vi "Begin.vi"(11 "Image Size":T1=enum."160x120") -> (0 "error out":errorcluster)   [LabVIEW 2011]
doc: "Called before other user functions, this VI is expected to open initial I/O refnums, load in file data, and do all program initialization. Notice that the <B>error out</B> terminal is simply used for data flow. Wiring it to other structures or subVIs ensures that this VI runs first."
uses:
  <vilib>/Rock Robotics/WPI/Camera/WPI_CameraImageSize.ctl
  <vilib>/Rock Robotics/WPI/Camera/WPI_CameraWhite Balance Values.ctl
  <vilib>/Rock Robotics/WPI/Camera/WPI_CameraExposure Values.ctl
  <vilib>/Rock Robotics/WPI/Camera/WPI_CameraFrameRate.ctl
  <vilib>/Rock Robotics/SystemInterfaces/DIO/FPGA_DIOPWMChannel.ctl
  <vilib>/Rock Robotics/SystemInterfaces/Typedef/FPGA_TypedefDigitalModule.ctl
  <vilib>/Rock Robotics/SystemInterfaces/DIO/FPGA_DIOChannel.ctl
  <vilib>/Rock Robotics/WPI/Encoder/WPI_EncoderType.ctl
  <vilib>/Rock Robotics/SystemInterfaces/Typedef/FPGA_TypedefAnalogModule.ctl
  <vilib>/Rock Robotics/SystemInterfaces/AI/FPGA_AIChannel.ctl
  <vilib>/Rock Robotics/SystemInterfaces/DIO/FPGA_DIORelayChannel.ctl
  <vilib>/Rock Robotics/WPI/Joystick/WPI_JoystickDeviceEnum.ctl
  <vilib>/Rock Robotics/WPI/RobotDrive/WPI_RobotDriveOpen4MotorWithVictor.vi
  <vilib>/Rock Robotics/WPI/MotorControl/WPI_MotorControlOpen Victor.vi
  <vilib>/Rock Robotics/WPI/Counter/WPI_CounterDigitalInputToDigitalSource.vi
panel:
  in  "Image Size 2":T1=enum."160x120"
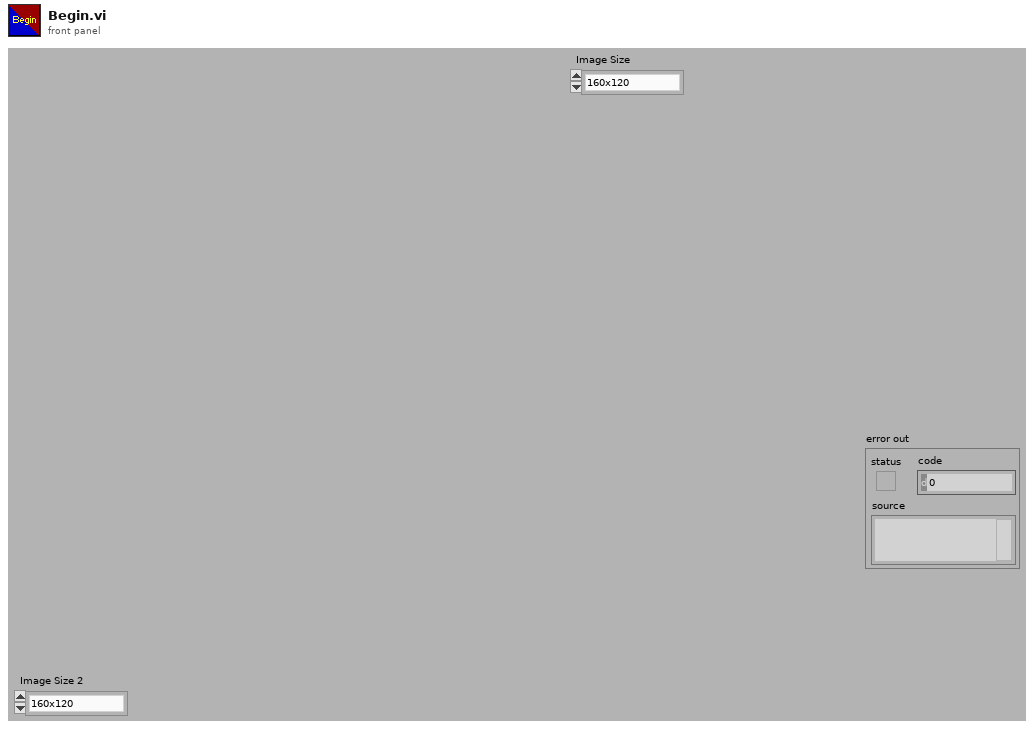
[diagram p1: front panel]
types:
  T1 = typedef "WPI_CameraImageSize.ctl" = enum16{"640x480", "320x240", "160x120"}
  T2 = typedef "FPGA_DIOChannel.ctl" = enum8{"DIO 1", "DIO 2", "DIO 3", "DIO 4", "DIO 5", "DIO 6", "DIO 7", "DIO 8", "DIO 9", "DIO 10", "DIO 11", "DIO 12", "DIO 13", "DIO 14", "Invalid"}
  T3 = typedef "FPGA_TypedefDigitalModule.ctl" = enum16{"Digital Module 1", "Digital Module 2"}
  T4 = typedef "FPGA_DIORelayChannel.ctl" = enum8{"Relay 1", "Relay 2", "Relay 3", "Relay 4", "Relay 5", "Relay 6", "Relay 7", "Relay 8", "Invalid"}
  T5 = typedef "WPI_JoystickDeviceEnum.ctl" = enum16{"USB 1", "USB 2", "USB 3", "USB 4", "Kinect 1", "Kinect 2"}
  T6 = typedef "FPGA_DIOPWMChannel.ctl" = enum8{"PWM 1", "PWM 2", "PWM 3", "PWM 4", "PWM 5", "PWM 6", "PWM 7", "PWM 8", "PWM 9", "PWM 10", "Invalid"}
  T7 = typedef "FPGA_AIChannel.ctl" = enum8{"AI 1", "AI 2", "AI 3", "AI 4", "AI 5", "AI 6", "AI 7", "AI 8", "Invalid"}
  T8 = typedef "FPGA_TypedefAnalogModule.ctl" = enum16{"Analog Module 1", "Analog Module 2"}
  T9 = typedef "WPI_EncoderType.ctl" = enum16{"1x", "2x", "4x"}
  T10 = typedef "WPI_CameraFrameRate.ctl" = u32
  T11 = typedef "WPI_CameraExposure Values.ctl" = enum16{"Auto", "Flicker-free 50 Hz", "Flicker-free 60 Hz", "Hold current"}
  T12 = typedef "WPI_CameraWhite Balance Values.ctl" = enum16{"Auto", "Fixed indoor", "Fixed outdoor 1", "Fixed outdoor 2", "Fixed fluorescent 1", "Fixed fluorescent 2", "Hold current"}
  T13 = typedef "WPI_MotorControlDeviceRef.ctl" = cluster{"DeviceStatus":errorcluster, "Type":enum16{"PWM", "CAN"}, "PWM":cluster{"Digital Module":T3, "PWM Channel":T6, "DeadBand":T14}, "CAN":cluster{"Device Number":u8, "Control Mode":T15, "Semaphore":T16, "Max Vout":dbl}, "Invert":bool, "TransformRef":T17, "InvTransformRef":T17}
  T14 = typedef "WPI_PWMDeadband.ctl" = cluster{"Name":string, "maxPositivePwm":i32, "minPositivePwm":i32, "centerPwm":i32, "maxNegativePwm":i32, "minNegativePwm":i32, "angularRange":u16}
  T15 = typedef "WPI_CANJaguar_ControlMode.ctl" = enum8{"Percent VBus", "Current", "Speed", "Position", "Voltage"}
  T16 = typedef "Semaphore RefNum" = refnum<k1>
  T17 = typedef "WPI_PWMTransform_ConPane.ctl" = refnum<vi>
  T18 = typedef "WPI_RobotDriveDevRef.ctl" = cluster{"DevStatus":errorcluster, "Motors[]":T13[], "Square Inputs":bool, "Max Output":dbl, "Isochronous":bool}
  T19 = typedef "WPI_CameraDevRef.ctl" = cluster{"Camera Address":string, "CameraStatus":errorcluster, "Acquire Image Notifier":refnum<notifier>}
  T20 = typedef "WPI_DigitalInputDevRef.ctl" = cluster{"DevStatus":errorcluster, "DIO Channel":T2, "Digital Module":T3}
  T21 = typedef "FPGA_CounterEncoderSourceConvertionLVSourceType.ctl" = cluster{"DevStatus":errorcluster, "AnalogTriggerMode?":bool, "DigitalMode":cluster{"Digital Module":T3, "DIO Channel":T22}, "AnalogTriggerMode":cluster{"AnalogTriggerIndex":T23, "OutputType":T24}}
  T22 = typedef "FPGA_DIODigitalSourceChannel.ctl" = enum8{"DIO 1", "DIO 2", "DIO 3", "DIO 4", "DIO 5", "DIO 6", "DIO 7", "DIO 8", "DIO 9", "DIO 10", "DIO 11", "DIO 12", "DIO 13", "DIO 14", "Disabled"}
  T23 = typedef "FPGA_AnalogTriggerIndex.ctl" = enum8{"Trig 0", "Trig 1", "Trig 2", "Trig 3", "Trig 4", "Trig 5", "Trig 6", "Trig 7", "Invalid"}
  T24 = typedef "FPGA_AnalogTriggerOutType.ctl" = enum16{"InWindow", "TriggerState", "Rising", "Falling"}
  T25 = typedef "WPI_AnalogChannelDevRef.ctl" = cluster{"DevStatus":errorcluster, "Analog Module":T8, "Analog Channel":T7}
  T26 = typedef "WPI_JoystickDevRef.ctl" = cluster{"Device":T5}
  T27 = typedef "WPI_RelayDevRef.ctl" = cluster{"DevStatus":errorcluster, "Relay Channel":T4, "Digital Module":T3, "Relay Direction":T28}
  T28 = typedef "WPI_RelayDirection.ctl" = enum16{"Both directions", "Forward only", "Reverse only"}
  T29 = typedef "WPI_EncoderDevRef.ctl" = cluster{"DevStatus":errorcluster, "EncoderIndex":T30, "CounterIndex":T31, "DistancePerCount":dbl, "Decoding Type":T9}
  T30 = typedef "FPGA_EncoderIdx.ctl" = enum8{"Enc 0", "Enc 1", "Enc 2", "Enc 3", "Invalid"}
  T31 = typedef "FPGA_CounterCtrSystemIndex.ctl" = enum8{"Ctr 0", "Ctr 1", "Ctr 2", "Ctr 3", "Ctr 4", "Ctr 5", "Ctr 6", "Ctr 7", "Invalid"}
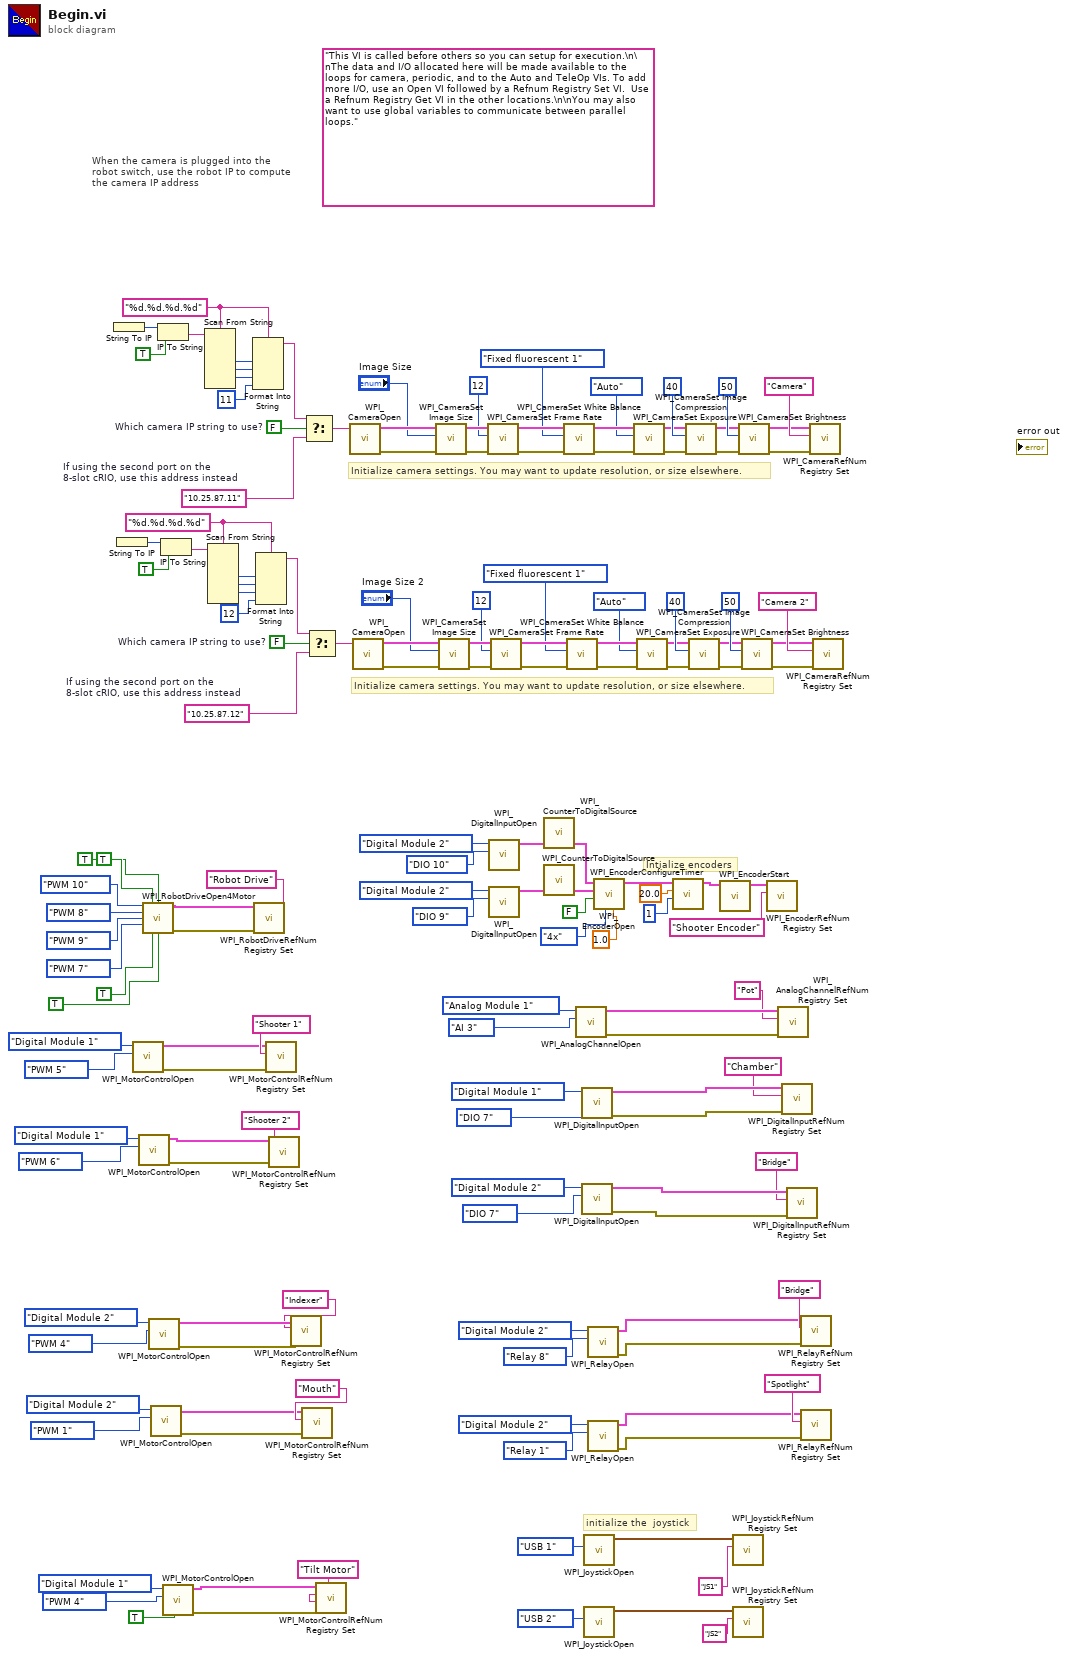
[diagram p0: block diagram]
diagram:
  w86 = FALSE  # Which camera IP string to use?
  w90 = "%d.%d.%d.%d" ("format string")
  w87 = "10.25.87.12"  # If using the second port on the 8-slot cRIO, use this address instead
  w119 = FALSE  # Which camera IP string to use?
  w123 = "%d.%d.%d.%d" ("format string")
  (unwired) "This VI is called before others so you can setup for execution.\n\nThe data and I/O allocated here will be made available to the loops for camera, periodic, and to the Auto and TeleOp VIs. To add more I/O, use an Open VI followed by a Refnum Registry Set VI.  Use a Refnum Registry Get VI in the other locations.\n\nYou may also want to use global variables to communicate between parallel loops."
  w120 = "10.25.87.11"  # If using the second port on the 8-slot cRIO, use this address instead
  # "initialize the  joystick"
  # "Intialize encoders"
  # "Initialize camera settings. You may want to update resolution, or size elsewhere."
  # "When the camera is plugged into the\nrobot switch, use the robot IP to compute\nthe camera IP address"
  # "Initialize camera settings. You may want to update resolution, or size elsewhere."
  n1 = String To IP() -> (0:w130:u32)  [unwired: 1 in]
  n2 = String To IP() -> (0:w97:u32)  [unwired: 1 in]
  n3 = call-poly <vilib>:"WPI_MotorControlOpen.vi"("PWM Channel"=FPGA_DIOPWMChannel."PWM 5", "Digital Module (Module 1)"=FPGA_TypedefDigitalModule."Digital Module 1") -> ("error out"=w69:errorcluster, "MotorControlDeviceRef"=w70:T13)  [unwired: 8 in]
  n4 = call-poly <vilib>:"WPI_MotorControlOpen.vi"("PWM Channel"=FPGA_DIOPWMChannel."PWM 6", "Digital Module (Module 1)"=FPGA_TypedefDigitalModule."Digital Module 1") -> ("error out"=w67:errorcluster, "MotorControlDeviceRef"=w68:T13)  [unwired: 8 in]
  n5 = call-poly <vilib>:"WPI_RobotDriveOpen4Motor.vi"("Rear Left Motor"=FPGA_DIOPWMChannel."PWM 10", "Rear Left Motor Inverted"=TRUE, "Rear Right Motor Inverted"=TRUE, "Rear Right Motor"=FPGA_DIOPWMChannel."PWM 8", "Front Left Motor"=FPGA_DIOPWMChannel."PWM 9", "Front Right Motor"=FPGA_DIOPWMChannel."PWM 7", "Front Left Motor Inverted"=TRUE, "Front Right Motor Inverted"=TRUE) -> ("RobotDriveDevRef"=w12:T18, "error out"=w11:errorcluster)  [unwired: 6 in]
  n6 = call-poly <vilib>:"WPI_MotorControlOpen.vi"("PWM Channel"=FPGA_DIOPWMChannel."PWM 4", "Digital Module (Module 1)"=FPGA_TypedefDigitalModule."Digital Module 2") -> ("error out"=w20:errorcluster, "MotorControlDeviceRef"=w21:T13)  [unwired: 8 in]
  n7 = call-poly <vilib>:"WPI_MotorControlOpen.vi"("PWM Channel"=FPGA_DIOPWMChannel."PWM 1", "Digital Module (Module 1)"=FPGA_TypedefDigitalModule."Digital Module 2") -> ("error out"=w62:errorcluster, "MotorControlDeviceRef"=w63:T13)  [unwired: 8 in]
  n8 = IP To String(1:TRUE ("dot notation? (F)"), 2:w130) -> (0:w128:string)
  n9 = IP To String(1:TRUE ("dot notation? (F)"), 2:w97) -> (0:w95:string)
  n10 = call-poly <vilib>:"WPI_MotorControlOpen.vi"("Invert"=TRUE, "PWM Channel"=FPGA_DIOPWMChannel."PWM 4", "Digital Module (Module 1)"=FPGA_TypedefDigitalModule."Digital Module 1") -> ("error out"=w56:errorcluster, "MotorControlDeviceRef"=w57:T13)  [unwired: 7 in]
  n11 = Scan From String(format string=w123, input string=w128) -> (output 1=w127:i32, output 2=w126:i32, output 3=w125:i32)  [unwired: 7 in, 3 out]
  n12 = Scan From String(format string=w90, input string=w95) -> (output 1=w94:i32, output 2=w93:i32, output 3=w92:i32)  [unwired: 7 in, 3 out]
  n13 = Format Into String(format string=w123, w127, w126, w125, 11 ("Compression")) -> (resulting string=w121:string)  [unwired: 2 in, 1 out]
  n14 = call <vilib>:"WPI_RobotDriveRefNum Registry Set.vi"("error in (no error)"=w11, "refnum name"="Robot Drive", "RobotDriveDevRef"=w12) -> ()  [unwired: 7 in, 2 out]
  n15 = Format Into String(format string=w90, w94, w93, w92, 12 ("Compression")) -> (resulting string=w88:string)  [unwired: 2 in, 1 out]
  n16 = call <vilib>:"WPI_MotorControlRefNum Registry Set.vi"("error in (no error)"=w69, "refnum name"="Shooter 1", "MotorControlDevRef"=w70) -> ()  [unwired: 7 in, 2 out]
  n17 = call <vilib>:"WPI_MotorControlRefNum Registry Set.vi"("error in (no error)"=w67, "refnum name"="Shooter 2", "MotorControlDevRef"=w68) -> ()  [unwired: 7 in, 2 out]
  n18 = call <vilib>:"WPI_MotorControlRefNum Registry Set.vi"("error in (no error)"=w20, "refnum name"="Indexer", "MotorControlDevRef"=w21) -> ()  [unwired: 7 in, 2 out]
  n19 = call <vilib>:"WPI_MotorControlRefNum Registry Set.vi"("error in (no error)"=w62, "refnum name"="Mouth", "MotorControlDevRef"=w63) -> ()  [unwired: 7 in, 2 out]
  n20 = Select(t=w121, s=w119, f=w120) -> (s? t:f=w122:string)
  n21 = Select(t=w88, s=w86, f=w87) -> (s? t:f=w89:string)
  n22 = call <vilib>:"WPI_MotorControlRefNum Registry Set.vi"("error in (no error)"=w56, "refnum name"="Tilt Motor", "MotorControlDevRef"=w57) -> ()  [unwired: 7 in, 2 out]
  n23 = call <vilib>:"WPI_CameraOpen.vi"("Camera Address"=w122) -> ("error out"=w142:errorcluster, "CameraDevRef"=w143:T19)  [unwired: 1 in, 8 out]
  n24 = call <vilib>:"WPI_CameraOpen.vi"("Camera Address"=w89) -> ("error out"=w109:errorcluster, "CameraDevRef"=w110:T19)  [unwired: 1 in, 8 out]
  n25 = call <vilib>:"WPI_CameraSet Image Size.vi"("error in (no error)"=w142, "Image Size"="Image Size", "CameraDevRef"=w143) -> ("error out"=w141:errorcluster, "CameraDevRef Out"=w144:T19)  [unwired: 7 out]
  n26 = call <vilib>:"WPI_CameraSet Image Size.vi"("error in (no error)"=w109, "Image Size"="Image Size 2", "CameraDevRef"=w110) -> ("error out"=w108:errorcluster, "CameraDevRef Out"=w111:T19)  [unwired: 7 out]
  n27 = call <vilib>:"WPI_CameraSet Frame Rate.vi"("error in (no error)"=w141, "Frame Rate (fps)"=T10 12, "CameraDevRef"=w144) -> ("error out"=w140:errorcluster, "CameraDevRef Out"=w146:T19)  [unwired: 7 out]
  n28 = call <vilib>:"WPI_DigitalInputOpen.vi"("DIO Channel"=FPGA_DIOChannel."DIO 10", "Digital Module (Module 1)"=FPGA_TypedefDigitalModule."Digital Module 2") -> ("DigitalInputDevRef"=w53:T20)  [unwired: 8 in, 1 out]
  n29 = call <vilib>:"WPI_DigitalInputOpen.vi"("DIO Channel"=FPGA_DIOChannel."DIO 9", "Digital Module (Module 1)"=FPGA_TypedefDigitalModule."Digital Module 2") -> ("DigitalInputDevRef"=w49:T20)  [unwired: 8 in, 1 out]
  n30 = call <vilib>:"WPI_CameraSet Frame Rate.vi"("error in (no error)"=w108, "Frame Rate (fps)"=T10 12, "CameraDevRef"=w111) -> ("error out"=w107:errorcluster, "CameraDevRef Out"=w113:T19)  [unwired: 7 out]
  n31 = call-poly <vilib>:"WPI_CounterToDigitalSource.vi"("DigitalInputDevRef"=w53) -> ("Digital Source"=w52:T21)  [unwired: 6 in]
  n32 = call-poly <vilib>:"WPI_CounterToDigitalSource.vi"("DigitalInputDevRef"=w49) -> ("Digital Source"=w48:T21)  [unwired: 6 in]
  n33 = call <vilib>:"WPI_CameraSet White Balance.vi"("error in (no error)"=w140, "White Balance"=WPI_CameraWhite_Balance_Values."Fixed fluorescent 1", "CameraDevRef"=w146) -> ("error out"=w139:errorcluster, "CameraDevRef Out"=w145:T19)  [unwired: 7 out]
  n34 = call <vilib>:"WPI_CameraSet White Balance.vi"("error in (no error)"=w107, "White Balance"=WPI_CameraWhite_Balance_Values."Fixed fluorescent 1", "CameraDevRef"=w113) -> ("error out"=w106:errorcluster, "CameraDevRef Out"=w112:T19)  [unwired: 7 out]
  n35 = call <vilib>:"WPI_AnalogChannelOpen.vi"("Analog Channel"=FPGA_AIChannel."AI 3", "Analog Module (Module 1)"=FPGA_TypedefAnalogModule."Analog Module 1") -> ("error out"=w34:errorcluster, "AIDeviceRef"=w36:T25)  [unwired: 8 in]
  n36 = call <vilib>:"WPI_DigitalInputOpen.vi"("DIO Channel"=FPGA_DIOChannel."DIO 7", "Digital Module (Module 1)"=FPGA_TypedefDigitalModule."Digital Module 1") -> ("error out"=w29:errorcluster, "DigitalInputDevRef"=w31:T20)  [unwired: 8 in]
  n37 = call <vilib>:"WPI_DigitalInputOpen.vi"("DIO Channel"=FPGA_DIOChannel."DIO 7", "Digital Module (Module 1)"=FPGA_TypedefDigitalModule."Digital Module 2") -> ("error out"=w1:errorcluster, "DigitalInputDevRef"=w3:T20)  [unwired: 8 in]
  n38 = call <vilib>:"WPI_JoystickOpen.vi"("JoystickDevice"=WPI_JoystickDeviceEnum."USB 1") -> ("JoystickDevRef"=w16:T26)  [unwired: 10 out]
  n39 = call <vilib>:"WPI_JoystickOpen.vi"("JoystickDevice"=WPI_JoystickDeviceEnum."USB 2") -> ("JoystickDevRef"=w15:T26)  [unwired: 10 out]
  n40 = call <vilib>:"WPI_RelayOpen.vi"("Relay Channel"=FPGA_DIORelayChannel."Relay 8", "Digital Module (Module 1)"=FPGA_TypedefDigitalModule."Digital Module 2") -> ("error out"=w6:errorcluster, "RelayDevRef"=w7:T27)  [unwired: 8 in]
  n41 = call <vilib>:"WPI_RelayOpen.vi"("Relay Channel"=FPGA_DIORelayChannel."Relay 1", "Digital Module (Module 1)"=FPGA_TypedefDigitalModule."Digital Module 2") -> ("error out"=w24:errorcluster, "RelayDevRef"=w25:T27)  [unwired: 8 in]
  n42 = call <vilib>:"WPI_EncoderOpen.vi"("DistancePerCount"=1.0, "Decoding Type"=WPI_EncoderType."4x", "Invert Direction (False)"=FALSE, "BSource"=w48, "ASource"=w52) -> ("EncoderDevRef"=w46:T29)  [unwired: 5 in, 1 out]
  n43 = call <vilib>:"WPI_CameraSet Exposure.vi"("error in (no error)"=w139, "Exposure"=WPI_CameraExposure_Values."Auto", "CameraDevRef"=w145) -> ("error out"=w138:errorcluster, "CameraDevRef Out"=w148:T19)  [unwired: 7 out]
  n44 = call <vilib>:"WPI_CameraSet Exposure.vi"("error in (no error)"=w106, "Exposure"=WPI_CameraExposure_Values."Auto", "CameraDevRef"=w112) -> ("error out"=w105:errorcluster, "CameraDevRef Out"=w115:T19)  [unwired: 7 out]
  n45 = call <vilib>:"WPI_EncoderConfigureTimer.vi"("Number Samples to Average"=u8 1, "Minimum Rate"=20.0, "EncoderDevRef"=w46) -> ("EncoderDevRef"=w40:T29)  [unwired: 7 in, 1 out]
  n46 = call <vilib>:"WPI_CameraSet Image Compression.vi"("error in (no error)"=w138, "Compression"=40, "CameraDevRef"=w148) -> ("error out"=w137:errorcluster, "CameraDevRef Out"=w147:T19)  [unwired: 7 out]
  n47 = call <vilib>:"WPI_CameraSet Image Compression.vi"("error in (no error)"=w105, "Compression"=40, "CameraDevRef"=w115) -> ("error out"=w104:errorcluster, "CameraDevRef Out"=w114:T19)  [unwired: 7 out]
  n48 = call <vilib>:"WPI_EncoderStart.vi"("EncoderDevRef"=w40) -> ("EncoderDevRef"=w39:T29)  [unwired: 9 in, 1 out]
  n49 = call <vilib>:"WPI_JoystickRefNum Registry Set.vi"("refnum name"="JS1", "JoystickDevRef"=w16) -> ()  [unwired: 1 in, 9 out]
  n50 = call <vilib>:"WPI_JoystickRefNum Registry Set.vi"("refnum name"="JS2", "JoystickDevRef"=w15) -> ()  [unwired: 1 in, 9 out]
  n51 = call <vilib>:"WPI_CameraSet Brightness.vi"("error in (no error)"=w137, "Brightness"=50, "CameraDevRef"=w147) -> ("error out"=w135:errorcluster, "CameraDevRef Out"=w136:T19)  [unwired: 7 out]
  n52 = call <vilib>:"WPI_CameraSet Brightness.vi"("error in (no error)"=w104, "Brightness"=50, "CameraDevRef"=w114) -> ("error out"=w102:errorcluster, "CameraDevRef Out"=w103:T19)  [unwired: 7 out]
  n53 = call <vilib>:"WPI_EncoderRefNum Registry Set.vi"("refnum name"="Shooter Encoder", "EncoderDevRef"=w39) -> ()  [unwired: 8 in, 2 out]
  n54 = call <vilib>:"WPI_AnalogChannelRefNum Registry Set.vi"("error in (no error)"=w34, "refnum name"="Pot", "AIDeviceRef"=w36) -> ()  [unwired: 7 in, 2 out]
  n55 = call <vilib>:"WPI_DigitalInputRefNum Registry Set.vi"("error in (no error)"=w29, "refnum name"="Chamber", "DigitalInputDevRef"=w31) -> ()  [unwired: 7 in, 2 out]
  n56 = call <vilib>:"WPI_DigitalInputRefNum Registry Set.vi"("error in (no error)"=w1, "refnum name"="Bridge", "DigitalInputDevRef"=w3) -> ()  [unwired: 7 in, 2 out]
  n57 = call <vilib>:"WPI_RelayRefNum Registry Set.vi"("error in (no error)"=w6, "refnum name"="Bridge", "RelayDevRef"=w7) -> ()  [unwired: 7 in, 2 out]
  n58 = call <vilib>:"WPI_RelayRefNum Registry Set.vi"("error in (no error)"=w24, "refnum name"="Spotlight", "RelayDevRef"=w25) -> ()  [unwired: 7 in, 2 out]
  n59 = call <vilib>:"WPI_CameraRefNum Registry Set.vi"("error in (no error)"=w135, "refnum name"="Camera", "CameraDevRef"=w136) -> ()  [unwired: 9 out]
  n60 = call <vilib>:"WPI_CameraRefNum Registry Set.vi"("error in (no error)"=w102, "refnum name"="Camera 2", "CameraDevRef"=w103) -> ()  [unwired: 9 out]
